vi "Create Arbitrary Waveform_Corr2.vi"(6 "Arbitrary Numeric Waveform Data":dbl[](array[numeric])=[1000.0, 2000.0, 3000.0, 4000.0, 5000.0, 6000.0, 7000.0, 8000.0], 8 "error in (no error)":errorcluster, 9 "Select Channel (1:Channel 1)":i32(ring)=1 items=["Channel 1"=1, "Channel 2"=2], 10 "Waveform Name (\"wave1\")":string="wave1", 11 "VISA resource name":refnum<visa-resource-name>="USB0::0xF4EC::0x1101::SDG6XEBC5R0119::INSTR") -> (0 "error out":errorcluster, 3 "VISA resource name out":refnum<visa-resource-name>)   [LabVIEW 2018]
doc: "Creates and saves an arbitrary (user-defined) waveform in non-volatile memory, then selects it for output."
panel:
  # "Same vi as with suppliers example,\nbut incorrect negativ case removed.\nInstead calculating twos complement\nexplicitly for negative values.\nThe input range for ARB data is\n-32768..+32767"
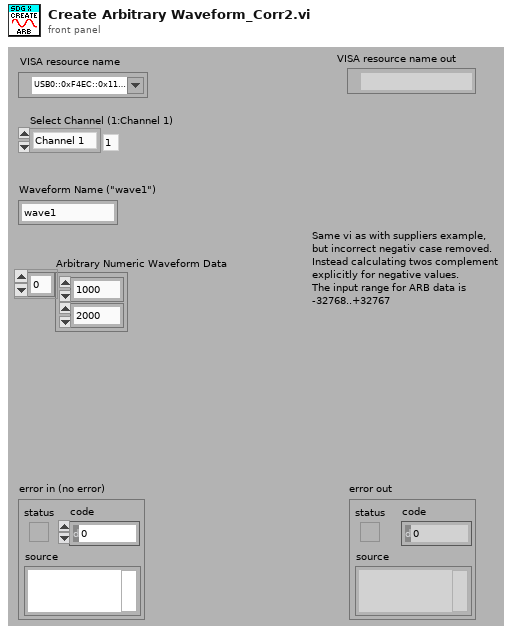
[diagram p1: front panel]
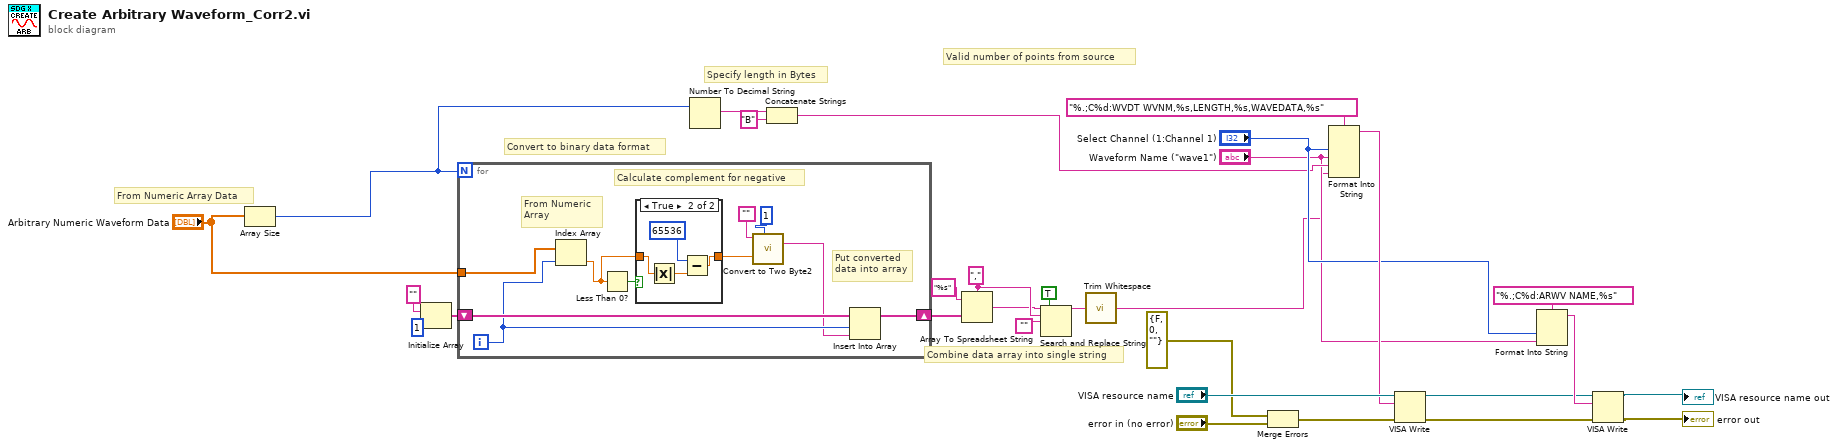
[diagram p0: block diagram]
diagram:
  w15 = ","
  # "From Numeric Array Data"
  # "Specify length in Bytes"
  # "Combine data array into single string"
  # "Valid number of points from source"
  # "Convert to binary data format"
  n1 = Array Size(array="Arbitrary Numeric Waveform Data") -> (size(s)=w23:i32)
  n2 = Initialize Array("", 1) -> (w19:string[])
  n3 = for {
    N: w23 -> [_]
    tunnel: "Arbitrary Numeric Waveform Data" -> [w38]
    shift-right: [w34] -> w6
    shift-left: w19 -> [w37]
    i -> [w36]
    # "Calculate complement for negative"
    # "From Numeric\nArray"
    # "Put converted\ndata into array"
    n4 = Index Array(array=w38, index=w36) -> (element=w32:dbl)
    n5 = Less Than 0?(x=w32) -> (x < 0?=w33:bool)
    n6 = case shown="True" w33 {
      tunnel: w32 -> [w41 w42]
      tunnel: [w41 w45] -> w31
      frame False {
      }
      frame True {
        n7 = Absolute Value(x=w42) -> (abs(x)=w43:dbl)
        n8 = Subtract(x=65536, y=w43) -> (x-y=w45:dbl)
      }
    }
    n9 = call "Convert to Two Byte2.vi"("Input Method (0:String)"=u16 1, "Input Number"=w31, "Numeric String"="") -> ("Output String"=w35:string)  [unwired: 8 in]
    n10 = Insert Into Array(array=w37, index=w36, new element=w35) -> (w34:string[])
  }
  n11 = Number To Decimal String(number=w23) -> (decimal integer string=w10:string)  [unwired: 1 in]
  n12 = Concatenate Strings(w10, "B" ("string")) -> (w8:string)
  n13 = Array To Spreadsheet String(delimiter (Tab)=w15, array=w6, 3:"%s") -> (spreadsheet string=w12:string)
  n14 = Search and Replace String(replace all?=TRUE, input string=w12, search string=w15, replace string="") -> (result string=w13:string)  [unwired: 4 in, 3 out]
  n15 = call <vilib>:"Trim Whitespace.vi"("string"=w13) -> ("trimmed string"=w1:string)  [unwired: 1 in]
  n16 = Merge Errors(errorcluster {"status"=FALSE, "code"=0, "source"=""} ("error constant"), "error in (no error)") -> (w25:errorcluster)
  n17 = Format Into String(format string="%.;C%d:WVDT WVNM,%s,LENGTH,%s,WAVEDATA,%s", "Select Channel (1:Channel 1)", "Waveform Name (\"wave1\")", w8, w1) -> (resulting string=w28:string)  [unwired: 2 in, 1 out]
  n18 = VISA Write(VISA resource name="VISA resource name", write buffer=w28, error in (no error)=w25) -> (VISA resource name out=w5:refnum<visa-resource-name>, error out=w4:errorcluster)  [unwired: 1 out]
  n19 = Format Into String(format string="%.;C%d:ARWV NAME,%s", "Select Channel (1:Channel 1)", "Waveform Name (\"wave1\")") -> (resulting string=w24:string)  [unwired: 2 in, 1 out]
  n20 = VISA Write(VISA resource name=w5, write buffer=w24, error in (no error)=w4) -> (VISA resource name out=→"VISA resource name out":refnum<visa-resource-name>, error out=→"error out":errorcluster)  [unwired: 1 out]
